vi "Save Active Chal.vi"(8 "error in (no error)":errorcluster, 10 "Active Chal":i64, 11 "SOL-Config in":refnum<class "SOL-Config.lvclass">) -> (0 "error out":errorcluster, 3 "SOL-Config out":refnum<class "SOL-Config.lvclass">)   [LabVIEW 2020, in "Summer of LabVIEW.lvlib" / "SOL-Config.lvclass"]
uses:
  SOL-Config.lvclass
  SOL-Config.lvclass/SOL-Config.ctl
  <vilib>/Utility/config.llb/NI_LVConfig.lvlib
  <vilib>/Utility/config.llb/Write Key (I32).vi
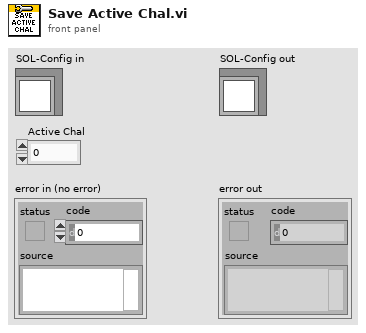
[diagram p1: front panel]
types:
  T1 = typedef "NI_LVConfig.lvlib/Config Data RefNum.ctl" = refnum<k1>
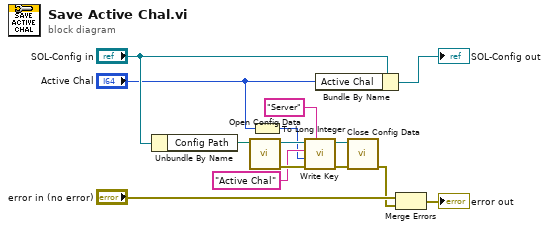
[diagram p0: block diagram]
diagram:
  n1 = Unbundle By Name("SOL-Config in") -> ("Config Path"=w11:path)
  n2 = call <vilib>:"Open Config Data.vi"("configuration file path"=w11) -> ("error out"=w9:errorcluster, "refnum"=w10:T1)  [unwired: 8 in, 1 out]
  n3 = To Long Integer(number="Active Chal") -> (32bit integer=w5:i32)
  n4 = call-poly <vilib>:"Write Key.vi"("section"="Server" ("key"), "error in (no error)"=w9, "value"=w5, "key"="Active Chal", "refnum"=w10) -> ("error out"=w3:errorcluster, "refnum out"=w4:T1)  [unwired: 4 in, 1 out]
  n5 = Bundle By Name(cluster="SOL-Config in", "Active Chal"="Active Chal") -> (→"SOL-Config out":refnum<class "SOL-Config.lvclass">)
  n6 = call <vilib>:"Close Config Data.vi"("error in (no error)"=w3, "refnum"=w4) -> ("error out"=w1:errorcluster)  [unwired: 8 in, 1 out]
  n7 = Merge Errors("error in (no error)", w1) -> (→"error out":errorcluster)
